vi "无损图层.vi"() -> ()   [LabVIEW 2018]
uses:
  <vilib>/vision/Image Controls.llb/Overlay Property.ctl
  <vilib>/vision/NI_Vision_Development_Module.lvlib
panel:
  out "error out":errorcluster
  out "Image 2":T1(plugin-control)
  out "Image":T1(plugin-control)
  in  "路径":path
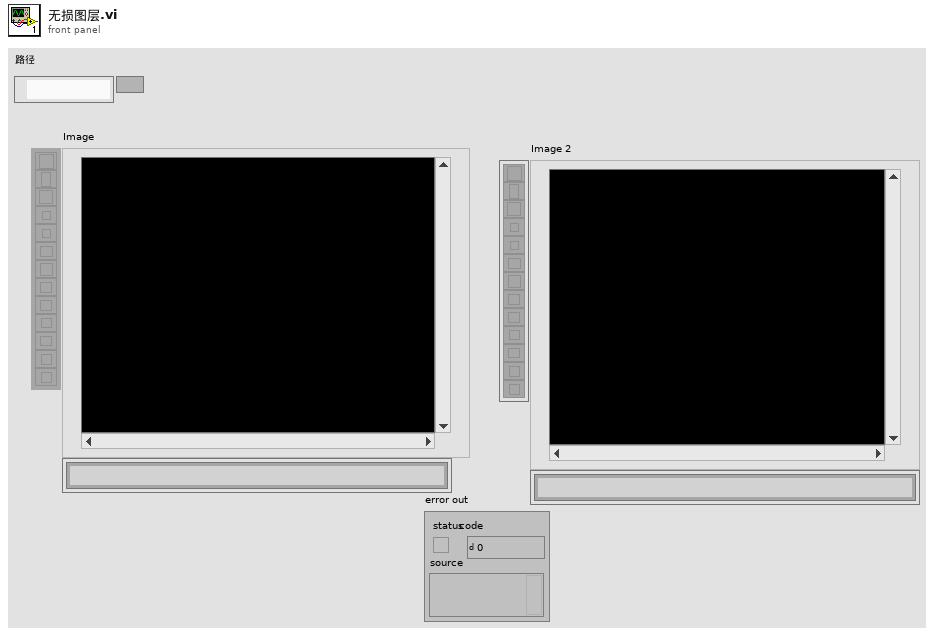
[diagram p1: front panel]
types:
  T1 = typedef "IMAQ Image.ctl" = refnum<image>
  T2 = typedef "Overlay Property.ctl" = cluster{"Property":enum32{"Scale", "Shift", "Rotate", "Symmetry"}, "Behavior":enum32{"Clear", "Keep", "Transform"}}
  T3 = cluster{"Area":dbl, "Number of Holes":dbl, "Bounding Rect":cluster{"Left":dbl, "Top":dbl, "Right":dbl, "Bottom":dbl}, "Center of Mass":cluster{"X":dbl, "Y":dbl}, "Orientation":dbl, "Dimensions":cluster{"Width":dbl, "Height":dbl}}[]
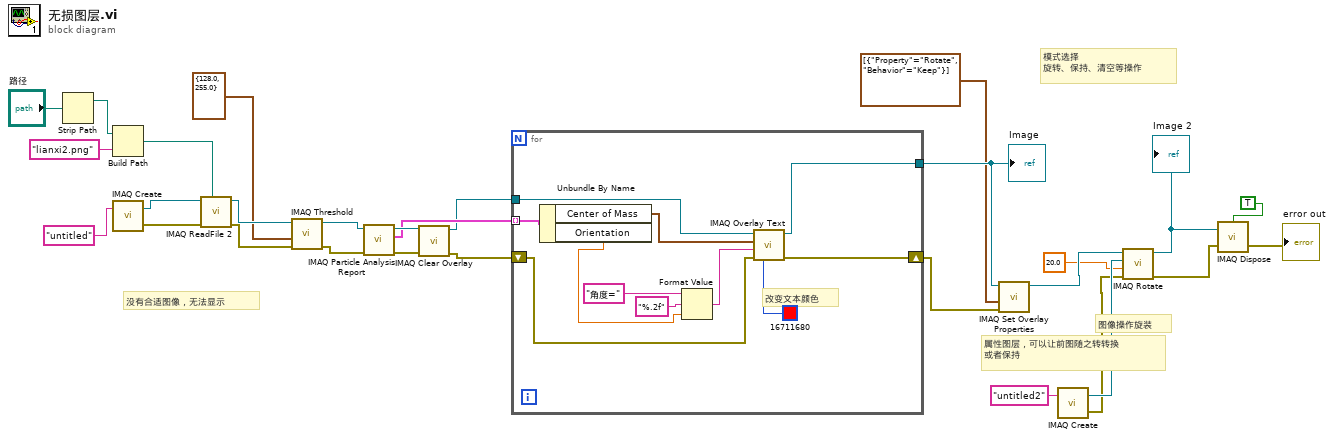
[diagram p0: block diagram]
diagram:
  # "没有合适图像，无法显示"
  # "模式选择\n旋转、保持、清空等操作"
  # "图像操作旋装"
  # "属性图层，可以让前图随之转转换\n或者保持"
  n1 = Strip Path(path="路径") -> (stripped path=w28:path)  [unwired: 1 out]
  n2 = Build Path(base path=w28, name or relative path="lianxi2.png" ("名称或相对路径")) -> (appended path=w23:path)
  n3 = call "IMAQ Create"("Image Name"="untitled") -> ("New Image"=w25:T1, "error out"=w24:errorcluster)  [unwired: 4 in]
  n4 = call "IMAQ ReadFile 2"("File Path"=w23, "error in (no error)"=w24, "Image"=w25) -> ("error out"=w19:errorcluster, "Image Out"=w20:T1)  [unwired: 4 in, 3 out]
  n5 = call "IMAQ Threshold"("error in (no error)"=w19, "Range"=cluster{"Lower value":sgl, "Upper value":sgl} {"Lower value"=128.0, "Upper value"=255.0}, "Image Src"=w20) -> ("error out"=w16:errorcluster, "Image Dst Out"=w17:T1)  [unwired: 7 in]
  n6 = call "IMAQ Particle Analysis Report"("error in (no error)"=w16, "Image"=w17) -> ("error out"=w14:errorcluster, "Particle Reports (Pixels)"=w13:T3, "Image Out (duplicate)"=w15:T1)  [unwired: 4 in, 3 out]
  n7 = call "IMAQ Clear Overlay"("error in (no error)"=w14, "Image"=w15) -> ("error out"=w12:errorcluster, "Image Out"=w11:T1)  [unwired: 8 in]
  n8 = for {
    tunnel: w13 -> [w40] mode=indexing
    shift-right: [w33] -> w4
    shift-left: w12 -> [w38]
    tunnel: w11 -> [w34]
    tunnel: [w32] -> w10
    # "改变文本颜色"
    n9 = Unbundle By Name(w40) -> ("Center of Mass"=w39:cluster{"X":dbl, "Y":dbl}, "Orientation"=w37:dbl)
    n10 = Format Value(string ("")="角度=" ("字符串(\"\")"), format string="%.2f" ("格式字符串"), value (0)=w37) -> (output string=w30:string)
    n11 = call "IMAQ Overlay Text"("Text Color (black)"=u32 16711680, "error in (no error)"=w38, "String"=w30, "Origin"=w39, "Image"=w34) -> ("error out"=w33:errorcluster, "Image Out"=w32:T1)  [unwired: 5 in]
  }
  "Image" <- w10
  n12 = call "IMAQ Set Overlay Properties"("Image"=w10, "Properties"=T2[] [{"Property"=enum."Rotate", "Behavior"=enum."Keep"}], "error in (no error)"=w4) -> ("Image Out"=w9:T1)  [unwired: 5 in, 1 out]
  n13 = call "IMAQ Create"("Image Name"="untitled2") -> ("New Image"=w7:T1, "error out"=w6:errorcluster)  [unwired: 4 in]
  n14 = call "IMAQ Rotate"("error in (no error)"=w6, "Angle (degrees)"=sgl 20.0, "Image Dst"=w7, "Image Src"=w9) -> ("error out"=w1:errorcluster, "Image Dst Out"=w2:T1)  [unwired: 6 in]
  "Image 2" <- w2
  n15 = call "IMAQ Dispose"("All Images? (No)"=TRUE, "Image"=w2, "error in (no error)"=w1) -> ("error out"=→"error out":errorcluster)  [unwired: 3 in]
